vi "MCCMSG Destroy Object.vi"(8 "error in (no error)":errorcluster, 11 "hMCCmsg":i32) -> (0 "error out":errorcluster)   [LabVIEW 2012, in "MultiClamp 700B Controls.lvlib" / "AxMultiClampMsg.lvlib"]
doc: "AXMCCMSG void WINAPI MCCMSG_DestroyObject(HMCCMSG hMCCmsg);"
uses:
  AxMultiClampMsg.lvlib
  AxMultiClampMsg.dll
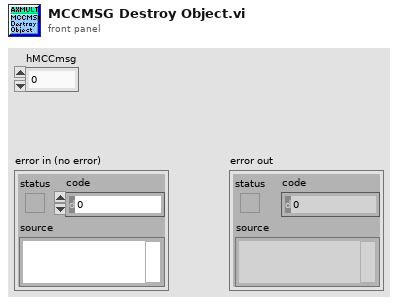
[diagram p1: front panel]
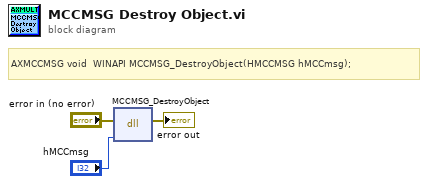
[diagram p0: block diagram]
diagram:
  # "AXMCCMSG void  WINAPI MCCMSG_DestroyObject(HMCCMSG hMCCmsg);"
  n1 = dll-call lib="C:/Users/Southampton/Desktop/Rita/Multiclamp 700B VIs/AxMultiClampMsg/AxMultiClampMsg.*" fn="MCCMSG_DestroyObject"(error in="error in (no error)", "hMCCmsg"="hMCCmsg") -> (error out=→"error out":errorcluster)  [unwired: 4 in, 1 out]
